vi "Decimate DFD (Decimation Factor).vi"(8 "error in (no error)":errorcluster, 10 "Decimation Factor":i32, 11 "Waveforms in":waveform(dbl)[](array[waveform])) -> (0 "error out":errorcluster, 3 "waveforms out":waveform(dbl)[](array[waveform]))   [LabVIEW 2019, in "Instrument.Lockin.lvlib" / "Instrument.DAQ.lvclass"]
uses:
  Instrument.DAQ.lvclass
  <vilib>/Analysis/2dsp.llb/Decimate (single shot, DBL).vi
  <vilib>/Analysis/NI_AALPro.lvlib
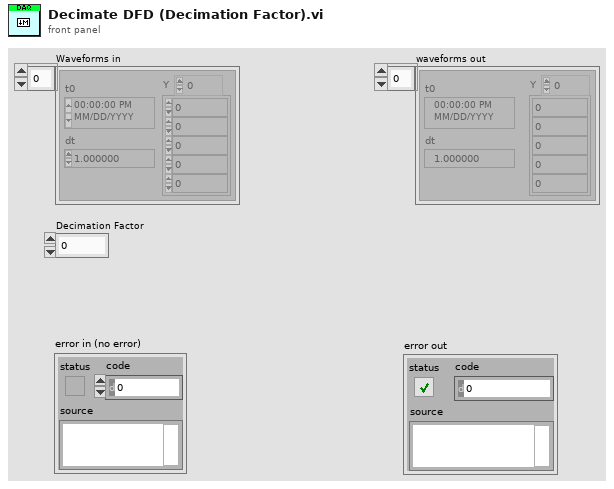
[diagram p1: front panel]
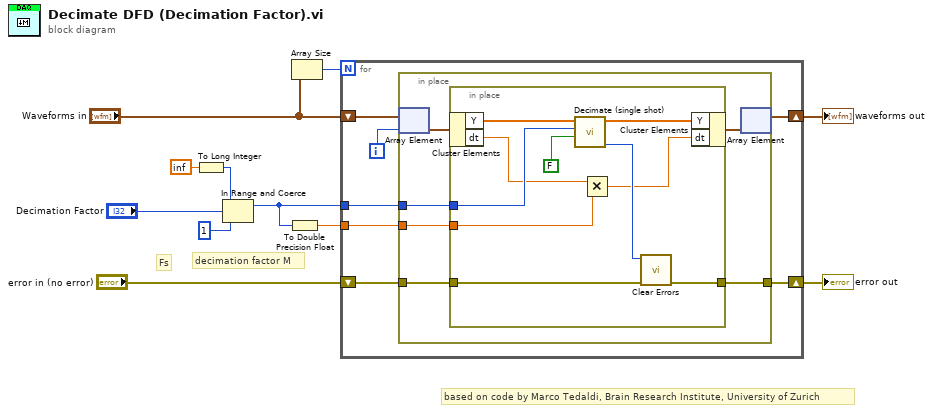
[diagram p0: block diagram]
diagram:
  # "based on code by Marco Tedaldi, Brain Research Institute, University of Zurich"
  # "Fs"
  # "decimation factor M"
  n1 = To Long Integer(number=inf) -> (32bit integer=w5:i32)
  n2 = In Range and Coerce(upper limit=w5, x="Decimation Factor", lower limit=1) -> (coerced(x)=w1:i32)  [unwired: 1 out]
  n3 = To Double Precision Float(number=w1) -> (double precision float=w2:dbl)
  n4 = Array Size(array="Waveforms in") -> (size(s)=w3:i32)
  n5 = for {
    N: w3 -> [_]
    tunnel: w2 -> [w18]
    shift-right: [w14] -> w11
    shift-left: "Waveforms in" -> [w16]
    tunnel: w1 -> [w13]
    shift-right: [w17] -> w9
    shift-left: "error in (no error)" -> [w12]
    i -> [w15]
    n6 = in-place {
      in-place-border: w18 -> [w23]
      in-place-border: [w24] -> w17
      in-place-border: w13 -> [w22]
      in-place-border: w12 -> [w21]
      n7 = in-place-array #1(w16, w15) -> (w20:waveform(dbl))
      n8 = in-place {
        in-place-border: [w34] -> w24
        in-place-border: w23 -> [w33]
        in-place-border: w22 -> [w32]
        in-place-border: w21 -> [w31]
        n9 = in-place-cluster #2(w20) -> ("Y"=w27:dbl[], "dt"=w28:dbl)
        n10 = call-poly <vilib>:"Decimate (single shot).vi"("averaging"=FALSE, "decimating factor"=w32, "X"=w27) -> ("error"=w30:i32, "Decimated Array"=w26:dbl[])  [unwired: 7 in]
        n11 = Multiply(x=w28, y=w33) -> (x*y=w25:dbl)
        n12 = call <vilib>:"Clear Errors.vi"("error in (no error)"=w31, "specific error code to clear (0: all)"=w30) -> ("error out"=w34:errorcluster)  [unwired: 4 in, 1 out]
        n13 = in-place-cluster #2("Y"=w26, "dt"=w25) -> (w19:waveform(dbl))
      }
      n14 = in-place-array #1(w19) -> (w14:waveform(dbl)[])  [unwired: 1 out]
    }
  }
  "waveforms out" <- w11
  "error out" <- w9
